vi "writeLogMessage.vi"(8 "error in (no error)":errorcluster, 10 "WriteLogMessageInput":T1, 11 "ITestLog in":refnum<class "ITestLog.lvclass">) -> (0 "error out":errorcluster, 3 "ITestLog out":refnum<class "ITestLog.lvclass">)   [LabVIEW 2015, in "ITestLog.lvclass"]
uses:
  ITestLog.lvclass
  Typedefs/WriteLogMessageInput.ctl
  Typedefs/FAMTTypedefs.lvlib
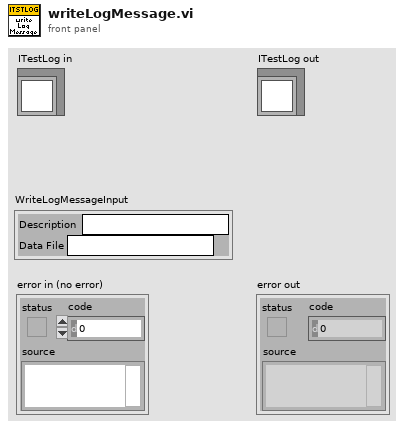
[diagram p1: front panel]
types:
  T1 = typedef "FAMTTypedefs.lvlib/WriteLogMessageInput.ctl" = cluster{"Description":string, "Data File":string}
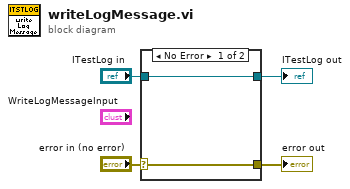
[diagram p0: block diagram]
diagram:
  n1 = case shown="No Error" "error in (no error)" {
    selector: "error in (no error)" -> [w5 w8]
    tunnel: [w5 w8] -> w3
    tunnel: [w6 w7] -> w1
    tunnel: "ITestLog in" -> [w6 w7]
    frame No Error {
    }
    frame Error {
    }
  }
  "error out" <- w3
  "ITestLog out" <- w1
